vi "SpecClose.vi"(3 "error in (no error)":errorcluster, 4 "队列":refnum<queue>, 5 "LightField Automation in":refnum<class "LightField Automation.lvclass">) -> (0 "error out":errorcluster)   [LabVIEW 2018]
uses:
  C:/ProgramData/Documents/Princeton Instruments/LightField/Add-in and Automation SDK/Samples/LabVIEW Automation/lightfield-automation-labview/LightField Automation.lvclass
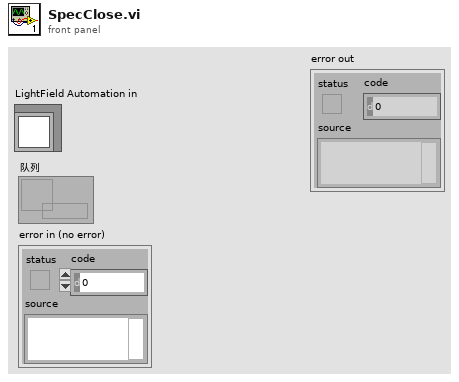
[diagram p1: front panel]
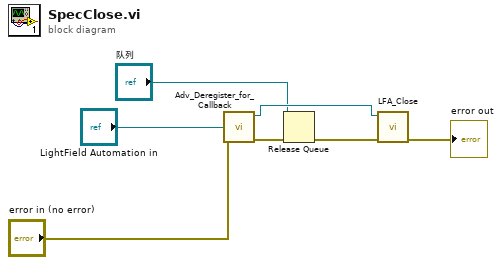
[diagram p0: block diagram]
diagram:
  n1 = call "Adv_Deregister_for_Callback.vi"("error in (no error)"="error in (no error)", "LightField Automation in"="LightField Automation in") -> ("error out"=w7:errorcluster, "LightField Automation out"=w6:refnum<class "LightField Automation.lvclass">)  [unwired: 8 in]
  n2 = Release Queue(queue="队列", error in (no error)=w7) -> (error out=w5:errorcluster)  [unwired: 1 in, 2 out]
  n3 = call "LFA_Close.vi"("error in (no error)"=w5, "LightField Automation in"=w6) -> ("error out"=→"error out":errorcluster)  [unwired: 8 in, 1 out]
